vi "SP_OEE_REPORT_DAYWISE.vi"() -> ()   [LabVIEW 2017]
uses:
  Controls/OE_screen_cluster.ctl
  <vilib>/addons/database/Connection.llb/Conn ObjectReference.ctl
  <vilib>/Utility/error.llb/DialogType.ctl
  <vilib>/addons/database/Connection.llb/DB Tools Open Connec (Path).vi
  <vilib>/addons/database/Connection.llb/Conn Execute.vi
  <vilib>/addons/database/Recordset.llb/Rec Fetch Recordset Data (R).vi
  <vilib>/addons/database/Recordset.llb/Rec Destroy - Connection.vi
  <vilib>/addons/database/NI_Database_API.lvlib
panel:
  in  "Tab Control 2":enum32{"Calculations", "Product Time"}(tab)
  out "AT time (Min)":i32
  out "Net Avai time (Min)":i32
  out "Standard DT (Min)":i32
  out "Downtime":u32
  out "Run Time":u32
  out "A Rate %":i32
  out "Parts per hours":i32
  out "CT":dbl format="%.2f"
  out "Actual Production / Total Quantity":u32
  out "Expected Run Time":sgl
  out "P Rate %":sgl format="%#.2g"
  out "OK Count":u32
  out "Rejection Count":u32
  out "Quality %":u32
  out "Select Product":string
  out "Start time":timestamp=timestamp(3772871939 s since 1904-01-01) format="%<%.X \n%x>T"
  out "End Time":timestamp=timestamp(3772871939 s since 1904-01-01) format="%<%.X \n%x>T"
  out "Split DT time":u32[](array[numeric])
  out "appended path":path
  in  "Reset":bool
  out "appended path 4":path
  out "OEE %":dbl format="%.2f"
  out "breakdown out time":string[](array[string])
  out "breakdown in time":string[](array[string])
  out "data":string[][](array[string])
  in  "shift time selection":enum32{"Shift 1", "Shift 2"}(tab)
  in  "mislanius times shift 1":T1={"Lunch Time\nFrom"=timestamp(3772871904 s since 1904-01-01), "Lunch Time To"=timestamp(3772871909 s since 1904-01-01), "Tea Time\nFrom"=timestamp(3772871914 s since 1904-01-01), "Tea Time To"=timestamp(3772871912 s since 1904-01-01), "Clean Time\nFrom"=timestamp(3772871918 s since 1904-01-01), "Clean Time To"=timestamp(3772871916 s since 1904-01-01), "Meeting Time\nFrom"=timestamp(3772871920 s since 1904-01-01), "Meeting Time To"=timestamp(3772871922 s since 1904-01-01), "Dev/Other Time\n From"=timestamp(3772871924 s since 1904-01-01), "Dev/Other Time To"=timestamp(3771057526 s since 1904-01-01), "Meeting"=FALSE, "Dev/Other"=TRUE} {"Dev/Other Time To" format="%<%.X\n %x>T"; "Dev/Other Time\n From" format="%<%.X\n %x>T"; "Meeting Time To" format="%<%.X\n %x>T"; "Meeting Time\nFrom" format="%<%.X\n %x>T"; "Clean Time To" format="%<%.X\n %x>T"; "Clean Time\nFrom" format="%<%.X\n %x>T"; "Tea Time To" format="%<%.X\n %x>T"; "Tea Time\nFrom" format="%<%.X\n %x>T"; "Lunch Time To" format="%<%.X\n %x>T"; "Lunch Time\nFrom" format="%<%.X\n %x>T"}
  in  "mislanius times shift 2":T2={"Dinner Time\nFrom"=timestamp(3772871937 s since 1904-01-01), "To"=timestamp(3772871939 s since 1904-01-01), "Tea Time\nFrom"=timestamp(3772958341 s since 1904-01-01), "Tea Time To"=timestamp(3772958344 s since 1904-01-01), "Clean Time\nFrom"=timestamp(3772871947 s since 1904-01-01), "Clean Time To"=timestamp(3772871950 s since 1904-01-01), "Meeting Time\nFrom"=timestamp(3772871952 s since 1904-01-01), "Meeting Time To"=timestamp(3772871954 s since 1904-01-01), "Dev/Other Time\nFrom"=timestamp(3772871934 s since 1904-01-01), "Dev/Other Time To"=timestamp(3772871932 s since 1904-01-01), "Meeting"=TRUE, "Dev/Other"=TRUE} {"Dev/Other Time To" format="%<%.X \n%x>T"; "Dev/Other Time\nFrom" format="%<%.X \n%x>T"; "Meeting Time To" format="%<%.X \n%x>T"; "Meeting Time\nFrom" format="%<%.X \n%x>T"; "Clean Time To" format="%<%.X \n%x>T"; "Clean Time\nFrom" format="%<%.X \n%x>T"; "Tea Time To" format="%<%.X \n%x>T"; "Tea Time\nFrom" format="%<%.X \n%x>T"; "To" format="%<%.X \n%x>T"; "Dinner Time\nFrom" format="%<%.X \n%x>T"}
  out "time stamp":timestamp[](array[timestamp])
  out "Part Per Hour":i16
  out "Plan data":string[][](array[string])
  in  "Select Product":string(combo)
  in  "Generate Report":bool
  out "error out 2":errorcluster
  in  "error in.":errorcluster
  in  "Home":bool
  in  "Date":timestamp format="%<%Y-%m-%d>T"
  in  "Shift":string(combo)
  in  "Tab Control":enum32{"Statistical", "Graphical"}(tab)
  in  "Select Station":string(combo)
  # "Date"
  # "Safety"
  # "Logistic"
  # "Maintenance"
  # "Quality"
  # "Production"
  # "Total"
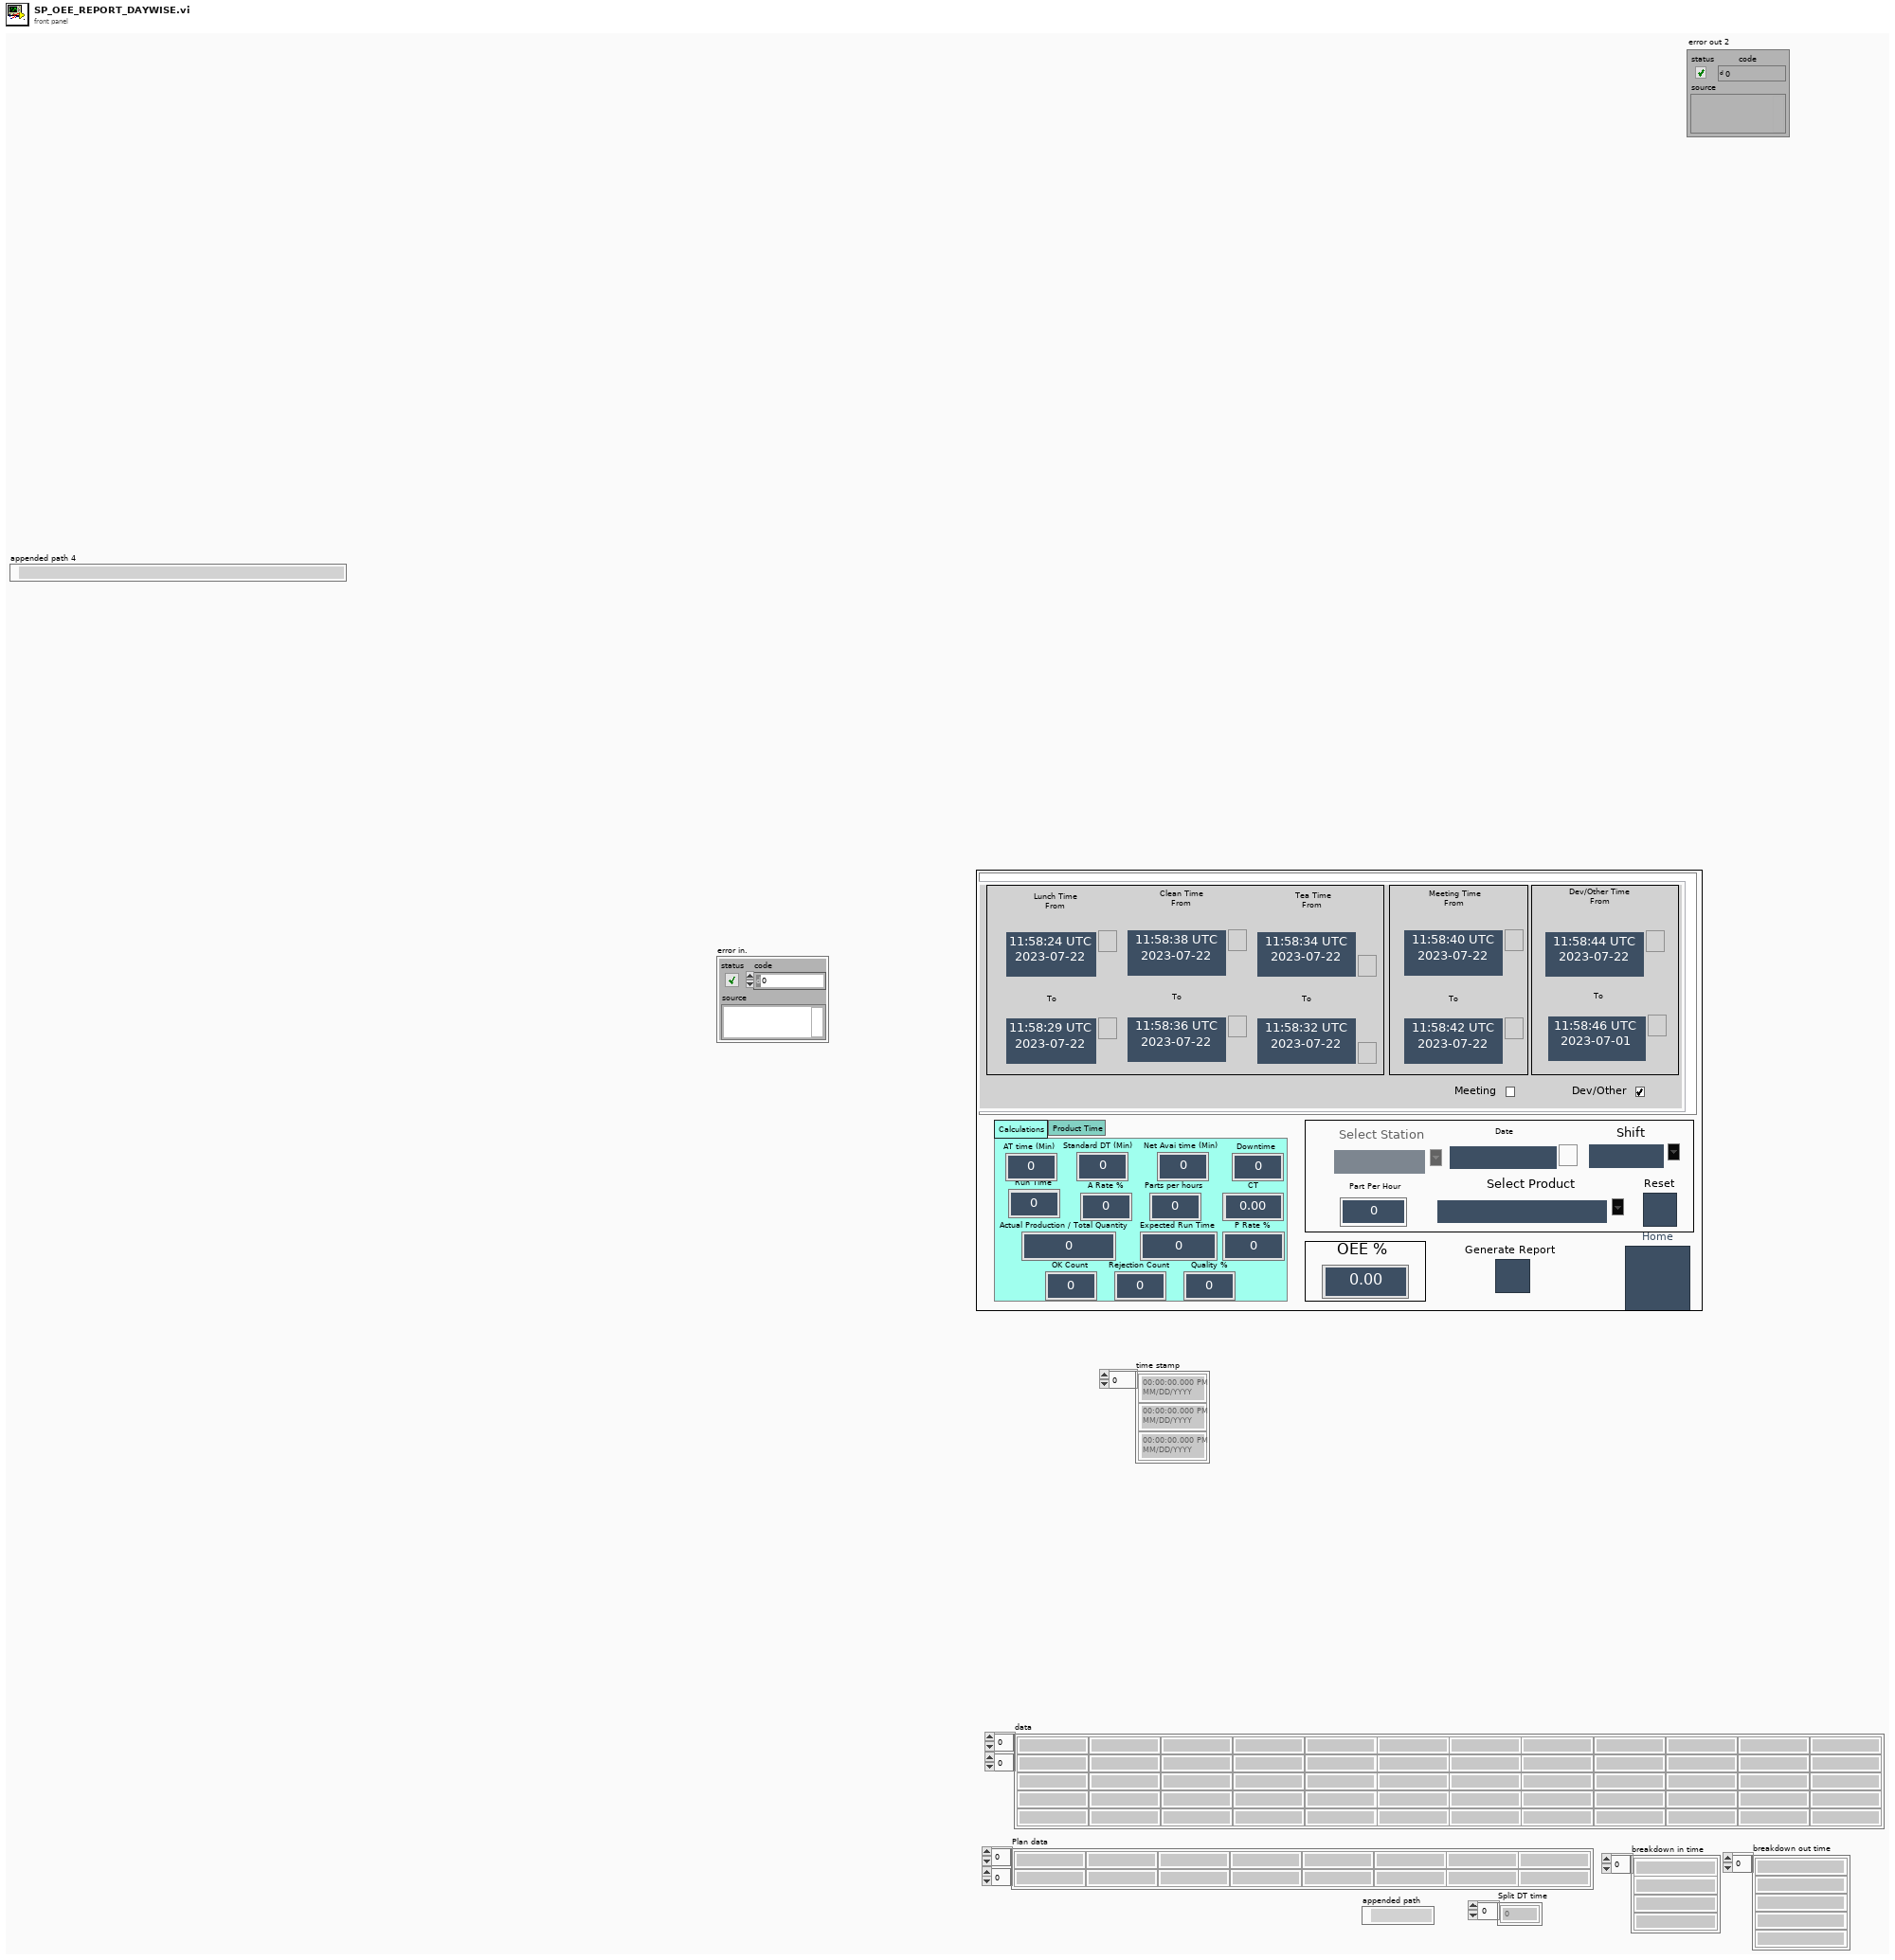
[diagram p1: front panel]
types:
  T1 = cluster{"Lunch Time\nFrom":timestamp, "Lunch Time To":timestamp, "Tea Time\nFrom":timestamp, "Tea Time To":timestamp, "Clean Time\nFrom":timestamp, "Clean Time To":timestamp, "Meeting Time\nFrom":timestamp, "Meeting Time To":timestamp, "Dev/Other Time\n From":timestamp, "Dev/Other Time To":timestamp, "Meeting":bool, "Dev/Other":bool}
  T2 = cluster{"Dinner Time\nFrom":timestamp, "To":timestamp, "Tea Time\nFrom":timestamp, "Tea Time To":timestamp, "Clean Time\nFrom":timestamp, "Clean Time To":timestamp, "Meeting Time\nFrom":timestamp, "Meeting Time To":timestamp, "Dev/Other Time\nFrom":timestamp, "Dev/Other Time To":timestamp, "Meeting":bool, "Dev/Other":bool}
  T3 = typedef "DialogType.ctl" = u16
  T4 = enum16{"open", "replace", "create", "open or create", "replace or create", "replace or create with confirmation"}
  T5 = cluster{"unsigned 64bit integer":u64, "unsigned 64bit integer 2":u64, "unsigned 64bit integer 3":u64, "unsigned 64bit integer 4":u64, "unsigned 64bit integer 5":u64, "unsigned 64bit integer 6":u64, "unsigned 64bit integer 7":u64, "unsigned 64bit integer 8":u64, "unsigned 64bit integer 9":u64, "unsigned 64bit integer 10":u64, "Meeting":bool, "Dev/other 1":bool, "unsigned 64bit integer 11":u64, "unsigned 64bit integer 12":u64, "unsigned 64bit integer 13":u64, "unsigned 64bit integer 14":u64, "unsigned 64bit integer 15":u64, "unsigned 64bit integer 16":u64, "unsigned 64bit integer 17":u64, "unsigned 64bit integer 18":u64, "unsigned 64bit integer 19":u64, "unsigned 64bit integer 20":u64, "Meeting 2":bool, "Dev/other 2":bool}
  T6 = enum8{"Enabled", "Disabled", "Disabled and Grayed Out"}
  T7 = typedef "OE_screen_cluster.ctl" = cluster{"connection reference":T8, "Net Avai time (Min)":i32, "pLAN dATE datA":string[][], "Data by plan date, shift, product":string[][], "BreakDownd Data":string[][], "Raw rejection Data":string[][], "mislanius times shift 1":cluster{"Lunch Time From":timestamp, "Lunch Time To":timestamp, "Tea Time From":timestamp, "Tea Time To":timestamp, "Clean Time From":timestamp, "Clean Time To":timestamp, "Meeting Time From":timestamp, "Meeting Time To":timestamp, "Dev/Other Time From":timestamp, "Dev/Other Time To":timestamp, "Meeting":bool, "Dev/Other":bool}, "mislanius times shift 2":cluster{"Lunch Time From":timestamp, "Lunch Time To":timestamp, "Tea Time From":timestamp, "Tea Time To":timestamp, "Clean Time From":timestamp, "Clean Time To":timestamp, "Meeting Time From":timestamp, "Meeting Time To":timestamp, "Dev/Other Time From":timestamp, "Dev/Other Time To":timestamp, "Meeting":bool, "Dev/Other":bool}}
  T8 = typedef "NI_Database_API.lvlib/Conn ObjectReference.ctl" = refnum<k1>
  T9 = enum32{"invalid app kind", "Development System", "Run Time System", "Student Edition", "Embedded LabVIEW", "Evaluation", "Custom"}
  T10 = typedef "NI_Database_API.lvlib/Rec ObjectReference.ctl" = refnum<k1>
  T11 = cluster{"delimiter (Tab)":string, "String":string}[]
  T12 = cluster{"Actual Production / Total Quantity":u32, "Part Per Hour":i16, "Rejection Count":u32}
  T13 = cluster{"Lunch Time From":timestamp, "Lunch Time To":timestamp, "Tea Time From":timestamp, "Tea Time To":timestamp, "Clean Time From":timestamp, "Clean Time To":timestamp, "Meeting Time From":timestamp, "Meeting Time To":timestamp, "Dev/Other Time From":timestamp, "Dev/Other Time To":timestamp, "Meeting":bool, "Dev/Other":bool}
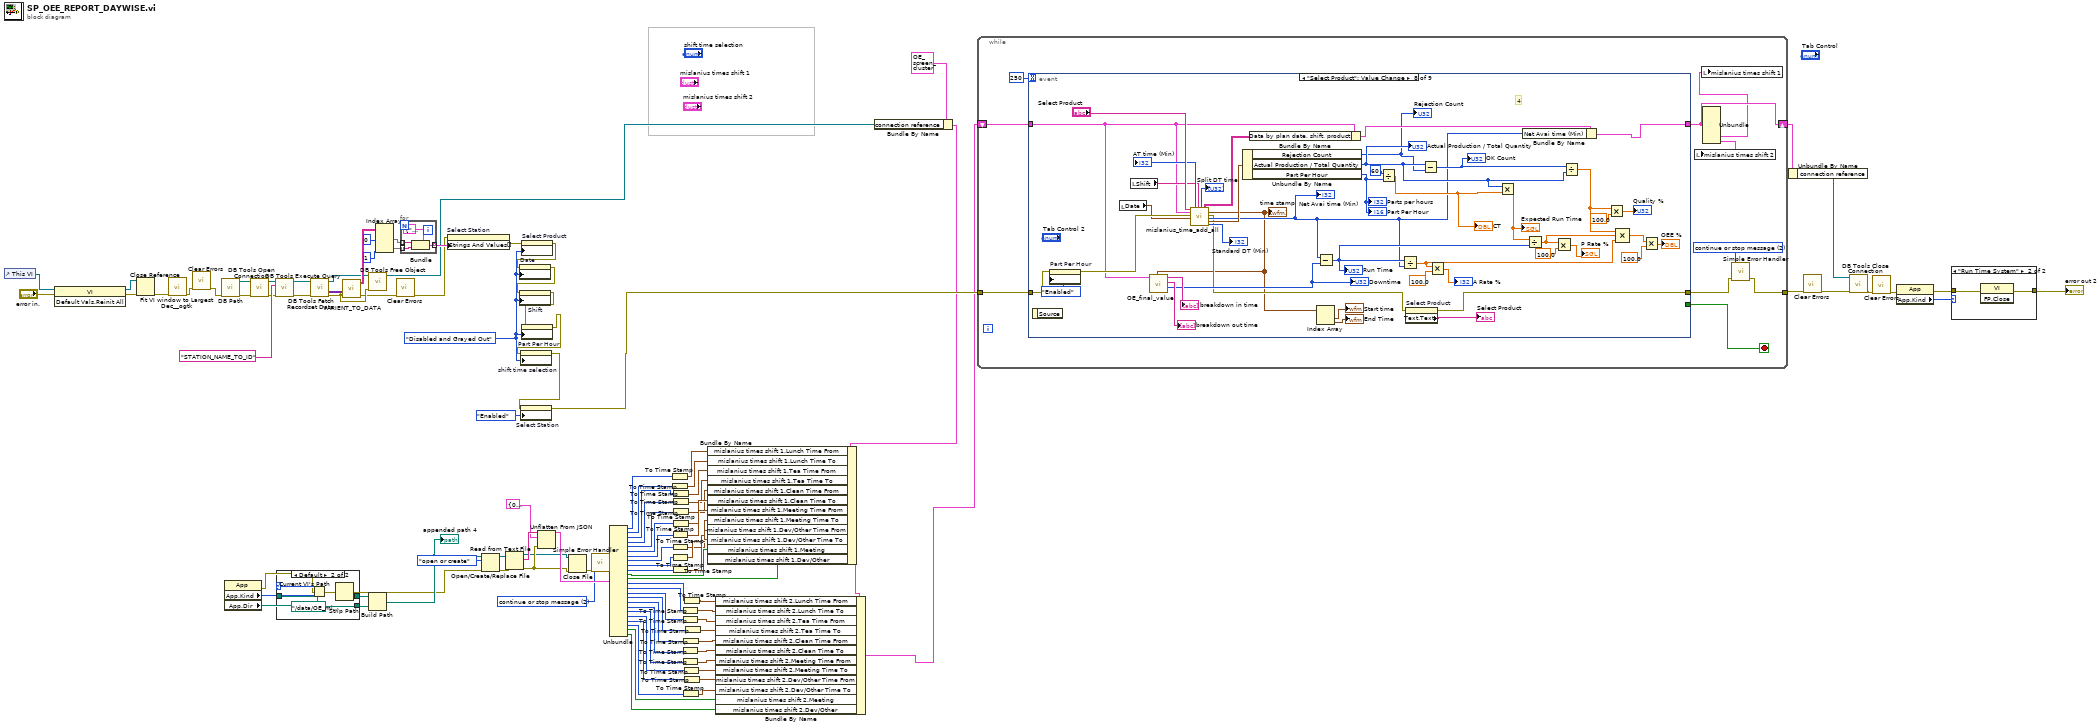
[diagram p0: block diagram]
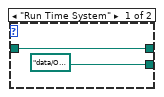
[diagram p2: hidden frame]
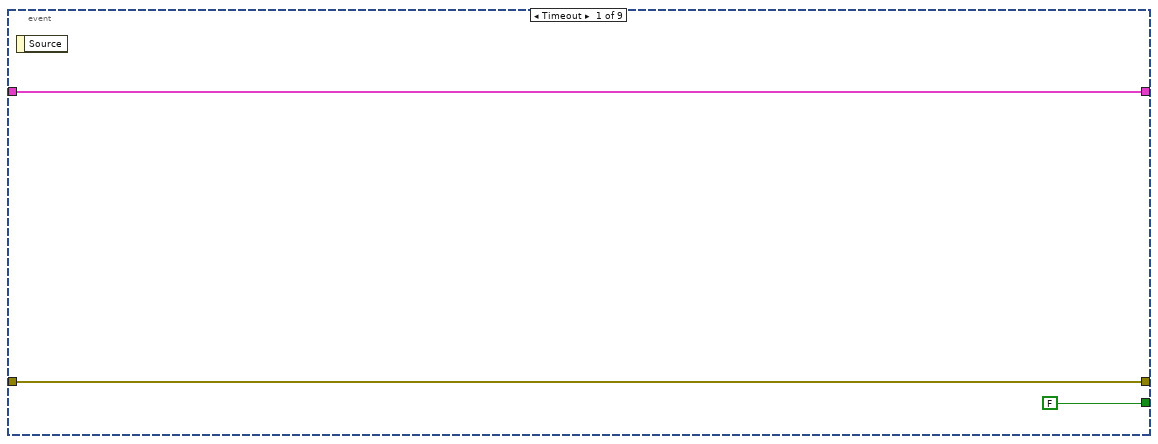
[diagram p4: hidden frame]
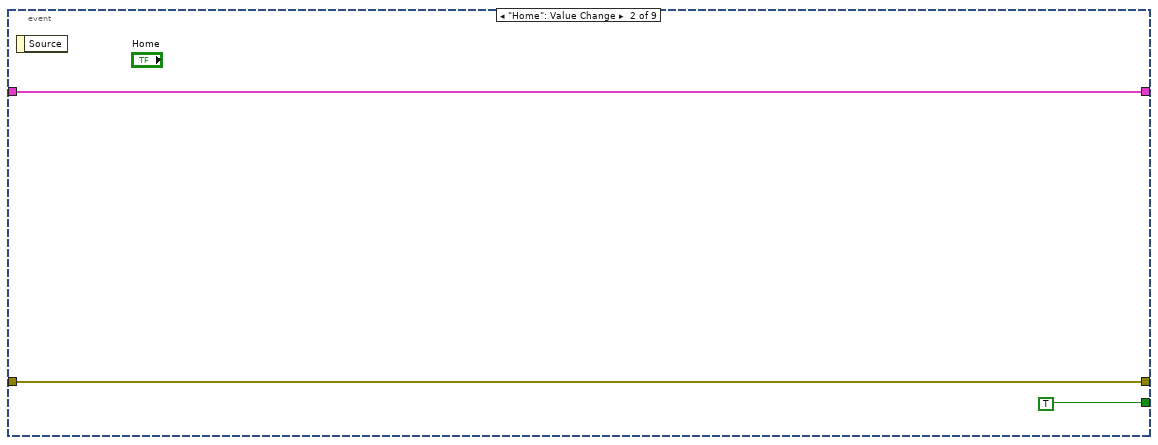
[diagram p5: hidden frame]
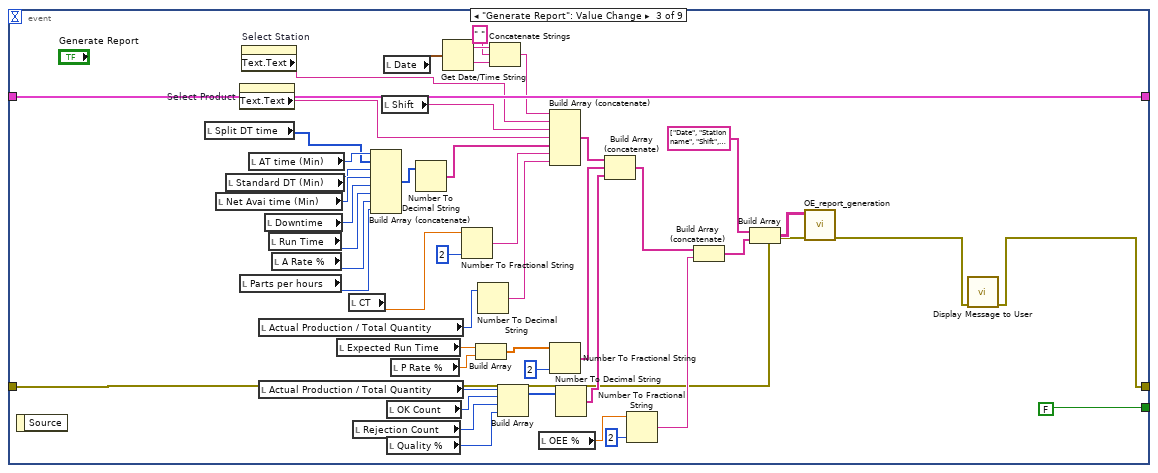
[diagram p6: hidden frame]
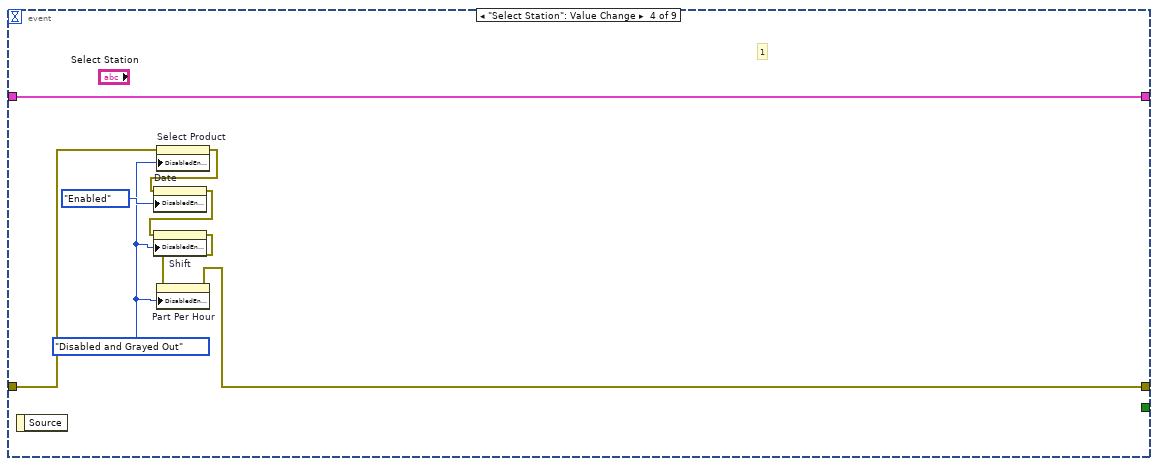
[diagram p7: hidden frame]
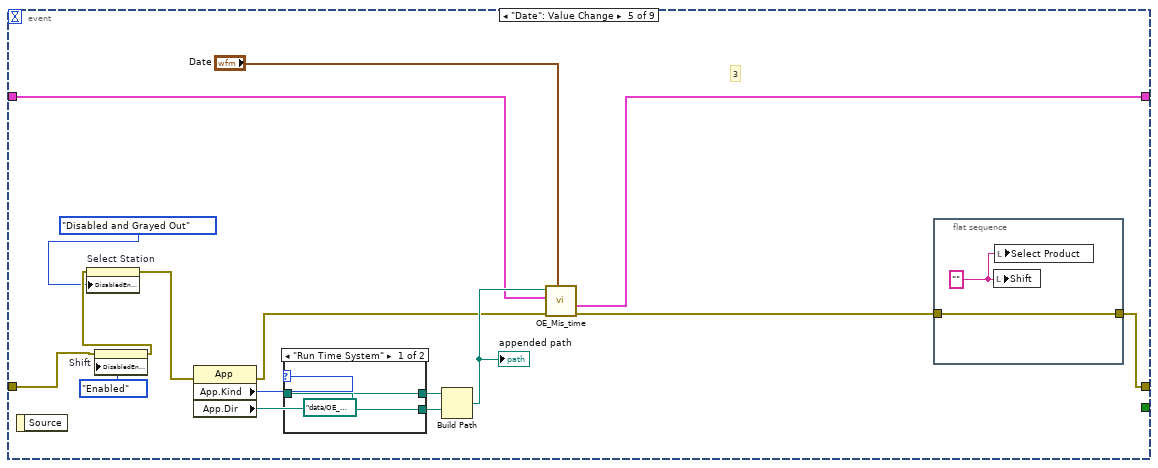
[diagram p8: hidden frame]
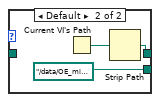
[diagram p9: hidden frame]
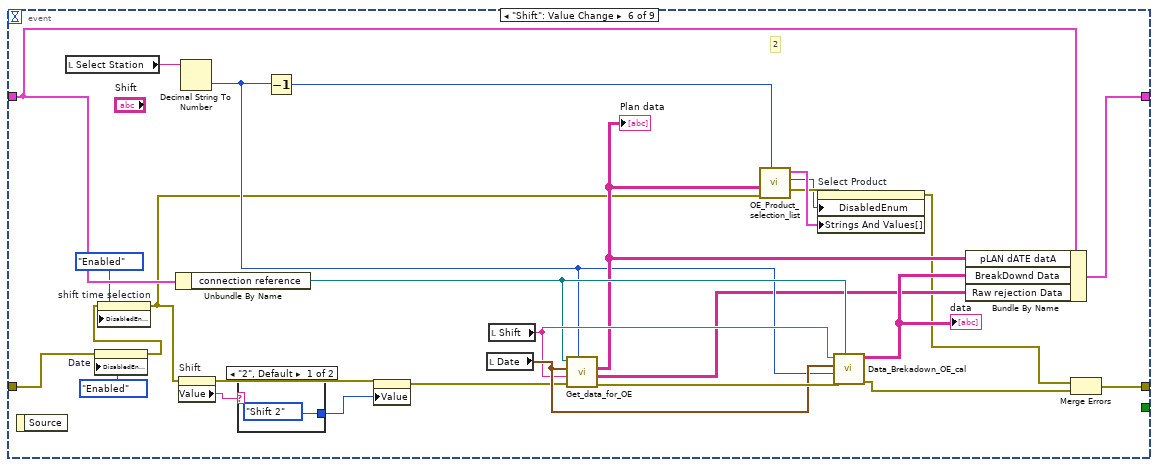
[diagram p10: hidden frame]
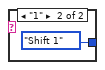
[diagram p11: hidden frame]
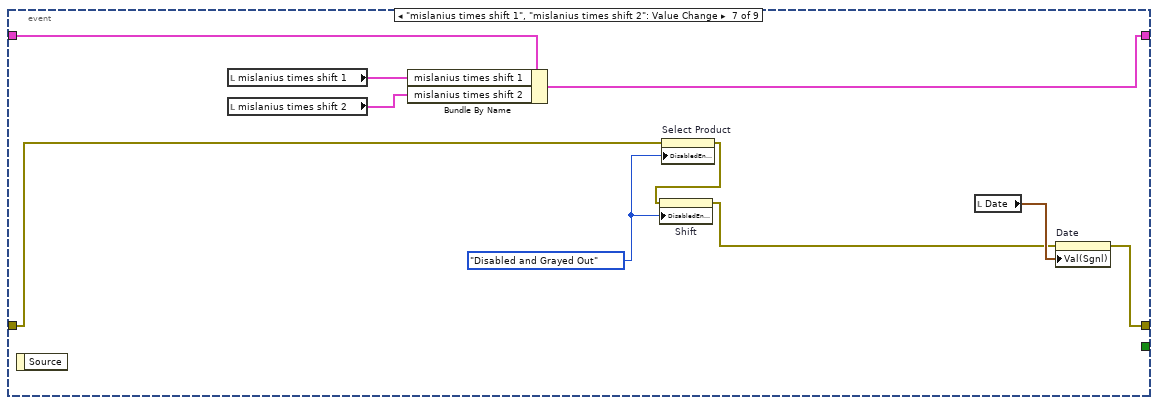
[diagram p12: hidden frame]
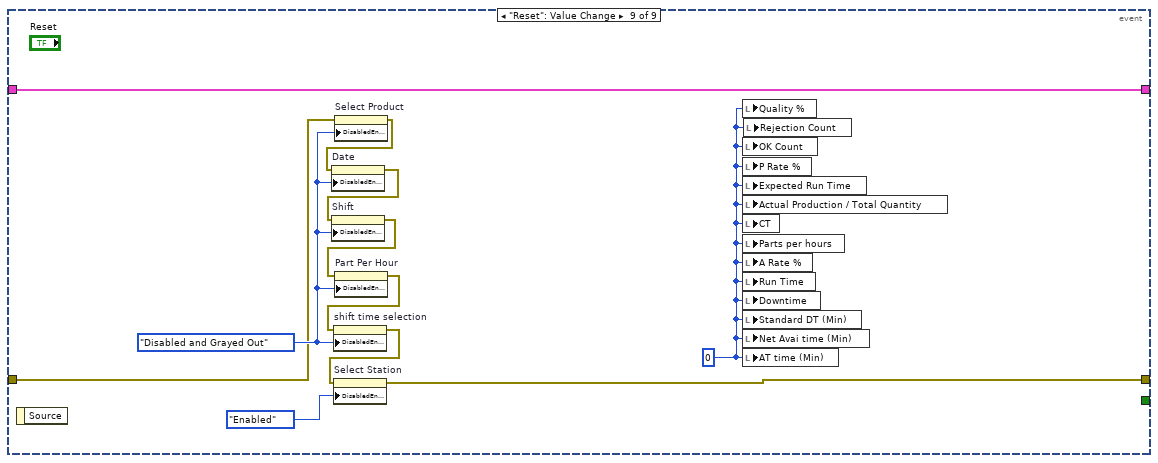
[diagram p13: hidden frame]
diagram:
  w6 = T3 2 items=["no dialog", "OK message", "continue or stop message", "OK message + warnings", "continue/stop + warnings"] ("type of dialog (OK msg:1)")
  w65 = T6."Disabled and Grayed Out" ("Disabled")
  n1 = control-ref of="This VI"() -> (w103:refnum<vi>)
  n2 = invoke class="VI" method="Default Vals.Reinit All"(reference=w103, error in="error in.") -> (reference out=w105:refnum<vi>, error out=w104:errorcluster)  [unwired: 1 in, 1 out]
  n3 = Close Reference(reference=w105, error in (no error)=w104) -> (error out=w5:errorcluster)
  n4 = call <userlib>:"Fit VI window to Largest Dec__ogtk.vi"("error in (no error)"=w5) -> ("error out"=w4:errorcluster)  [unwired: 5 in, 1 out]
  n5 = call <vilib>:"Clear Errors.vi"("error in (no error)"=w4) -> ("error out"=w3:errorcluster)  [unwired: 5 in, 1 out]
  n6 = call "DB Path.vi"("error in"=w3) -> ("error out"=w106:errorcluster, "DB Path"=w107:path)  [unwired: 9 in]
  n7 = property class="App"() -> (error out=w13:errorcluster, "App.Kind"=w70:T9, "App.Dir"=w71:path)  [unwired: 2 in, 1 out]
  n8 = call-poly <vilib>:"DB Tools Open Connection.vi"("error in (no error)"=w106, "connection information"=w107) -> ("error out"=w93:errorcluster, "connection reference"=w80:T8)  [unwired: 6 in]
  n9 = call-poly <vilib>:"DB Tools Execute Query.vi"("error in (no error)"=w93, "SQL query"="STATION_NAME_TO_ID", "connection reference"=w80) -> ("error out"=w101:errorcluster, "recordset reference"=w102:T10)  [unwired: 5 in]
  n10 = case shown="Default" w70 {
    tunnel: w71 -> [w110 _]
    tunnel: [path "data/OE_mis_time.txt" ("path") path "../data/OE_mis_time.txt" ("path")] -> w73
    tunnel: [w110 w112] -> w74
    frame "Run Time System" {
    }
    frame Default {
      n11 = Current VI's Path() -> (path=w113:path)
      n12 = Strip Path(path=w113) -> (stripped path=w112:path)  [unwired: 1 out]
    }
  }
  n13 = call-poly <vilib>:"DB Tools Fetch Recordset Data.vi"("error in (no error)"=w101, "recordset reference"=w102) -> ("error out"=w95:errorcluster, "recordset data"=w99:variant[][], "recordset reference out"=w81:T10)  [unwired: 3 in]
  n14 = call "VARIENT_TO_DATA.vi"("data"=w99, "error in (no error)"=w95) -> ("Table"=w96:string[][], "error out"=w94:errorcluster)  [unwired: 7 in]
  n15 = Build Path(base path=w74, name or relative path=w73) -> (appended path=w72:path)
  "appended path 4" <- w72
  n16 = call-poly <vilib>:"DB Tools Free Object.vi"("error in (no error)"=w95, "recordset reference"=w81) -> ("connection reference"=w79:T8)  [unwired: 8 in, 1 out]
  n17 = Index Array(array=w96, index (col) #1=0 ("index (row)"), index (col) #2=1 ("index (col)")) -> (element #1=w92:string[], element #2=w91:string[])  [unwired: 2 in]
  n18 = call <vilib>:"Clear Errors.vi"("error in (no error)"=w94) -> ("error out"=w89:errorcluster)  [unwired: 5 in, 1 out]
  n19 = for {
    tunnel: w92 -> [w117] mode=indexing
    tunnel: w91 -> [w116] mode=indexing
    tunnel: [w114] -> w90 mode=indexing
    n20 = Bundle(cluster=cluster{"String":string, "Value":string} {"String"="", "Value"=""}, "String"=w117, "Value"=w116) -> (w114:cluster{"String":string, "Value":string})
  }
  n21 = property on="Select Station" class="CmbBox"(error in=w89, "Strings And Values[]"=w90) -> (error out=w77:errorcluster)  [unwired: 1 in, 1 out]
  n22 = Open/Create/Replace File(file path (use dialog)=w72, error in=w13, operation (0:open)=T4."open or create") -> (refnum out=w69:refnum<file>, error out=w68:errorcluster)  [unwired: 3 in, 1 out]
  n23 = Read from Text File(file (use dialog)=w69, error in=w68) -> (refnum out=w9:refnum<file>, text=w12:string, error out=w10:errorcluster)  [unwired: 2 in, 1 out]
  n24 = property on="Select Product" class="CmbBox"(error in=w77, "DisabledEnum"=w65) -> (error out=w76:errorcluster)  [unwired: 1 in, 1 out]
  n25 = property on="Date" class="AbsTime (strict)"(error in=w76, "DisabledEnum"=w65) -> (error out=w78:errorcluster)  [unwired: 1 in, 1 out]
  n26 = property on="Shift" class="CmbBox"(error in=w78, "DisabledEnum"=w65) -> (error out=w75:errorcluster)  [unwired: 1 in, 1 out]
  n27 = property on="Part Per Hour" class="DigNum (strict)"(error in=w75, "DisabledEnum"=w65) -> (error out=w66:errorcluster)  [unwired: 1 in, 1 out]
  n28 = property on="shift time selection" class="TabCtl (strict)"(error in=w66, "DisabledEnum"=w65) -> (error out=w64:errorcluster)  [unwired: 1 in, 1 out]
  n29 = property on="Select Station" class="CmbBox"(error in=w64, "DisabledEnum"=T6."Enabled" ("Disabled")) -> (error out=w63:errorcluster)  [unwired: 1 in, 1 out]
  n30 = Unflatten From JSON(JSON string=w12, type and defaults=T5 {"unsigned 64bit integer"=0, "unsigned 64bit integer 2"=0, "unsigned 64bit integer 3"=0, "unsigned 64bit integer 4"=0, "unsigned 64bit integer 5"=0, "unsigned 64bit integer 6"=0, "unsigned 64bit integer 7"=0, "unsigned 64bit integer 8"=0, "unsigned 64bit integer 9"=0, "unsigned 64bit integer 10"=0, "Meeting"=FALSE, "Dev/other 1"=FALSE, "unsigned 64bit integer 11"=0, "unsigned 64bit integer 12"=0, "unsigned 64bit integer 13"=0, "unsigned 64bit integer 14"=0, "unsigned 64bit integer 15"=0, "unsigned 64bit integer 16"=0, "unsigned 64bit integer 17"=0, "unsigned 64bit integer 18"=0, "unsigned 64bit integer 19"=0, "unsigned 64bit integer 20"=0, "Meeting 2"=FALSE, "Dev/other 2"=FALSE} ("input cluster"), error in (no error)=w10) -> (value=w51:T5)  [unwired: 4 in, 1 out]
  n31 = Close File(refnum=w9, error in=w10) -> (error out=w7:errorcluster)  [unwired: 1 out]
  n32 = call <vilib>:"Simple Error Handler.vi"("type of dialog (OK msg:1)"=w6, "error in (no error)"=w7) -> ()  [unwired: 3 in, 5 out]
  n33 = Unbundle(w51) -> ("unsigned 64bit integer"=w36:u64, "unsigned 64bit integer 2"=w35:u64, "unsigned 64bit integer 3"=w34:u64, "unsigned 64bit integer 4"=w33:u64, "unsigned 64bit integer 5"=w32:u64, "unsigned 64bit integer 6"=w31:u64, "unsigned 64bit integer 7"=w30:u64, "unsigned 64bit integer 8"=w29:u64, "unsigned 64bit integer 9"=w28:u64, "unsigned 64bit integer 10"=w27:u64, "Meeting"=w38:bool, "Dev/other 1"=w37:bool, "unsigned 64bit integer 11"=w16:u64, "unsigned 64bit integer 12"=w17:u64, "unsigned 64bit integer 13"=w18:u64, "unsigned 64bit integer 14"=w19:u64, "unsigned 64bit integer 15"=w20:u64, "unsigned 64bit integer 16"=w21:u64, "unsigned 64bit integer 17"=w22:u64, "unsigned 64bit integer 18"=w23:u64, "unsigned 64bit integer 19"=w24:u64, "unsigned 64bit integer 20"=w25:u64, "Meeting 2"=w26:bool, "Dev/other 2"=w39:bool)
  n34 = To Time Stamp(1:w36) -> (0:w52:timestamp)
  n35 = To Time Stamp(1:w35) -> (0:w53:timestamp)
  n36 = To Time Stamp(1:w30) -> (0:w58:timestamp)
  n37 = To Time Stamp(1:w29) -> (0:w59:timestamp)
  n38 = To Time Stamp(1:w28) -> (0:w60:timestamp)
  n39 = To Time Stamp(1:w27) -> (0:w61:timestamp)
  n40 = To Time Stamp(1:w34) -> (0:w54:timestamp)
  n41 = To Time Stamp(1:w33) -> (0:w55:timestamp)
  n42 = To Time Stamp(1:w32) -> (0:w56:timestamp)
  n43 = To Time Stamp(1:w31) -> (0:w57:timestamp)
  n44 = To Time Stamp(1:w17) -> (0:w49:timestamp)
  n45 = To Time Stamp(1:w18) -> (0:w48:timestamp)
  n46 = To Time Stamp(1:w21) -> (0:w45:timestamp)
  n47 = To Time Stamp(1:w22) -> (0:w44:timestamp)
  n48 = To Time Stamp(1:w20) -> (0:w46:timestamp)
  n49 = To Time Stamp(1:w25) -> (0:w41:timestamp)
  n50 = To Time Stamp(1:w23) -> (0:w43:timestamp)
  n51 = To Time Stamp(1:w16) -> (0:w50:timestamp)
  n52 = To Time Stamp(1:w24) -> (0:w42:timestamp)
  n53 = To Time Stamp(1:w19) -> (0:w47:timestamp)
  n54 = Bundle By Name(cluster=T7 {"connection reference"=refnum, "Net Avai time (Min)"=0, "pLAN dATE datA"=[], "Data by plan date, shift, product"=[], "BreakDownd Data"=[], "Raw rejection Data"=[], "mislanius times shift 1"={"Lunch Time From"=timestamp(0 s since 1904-01-01), "Lunch Time To"=timestamp(0 s since 1904-01-01), "Tea Time From"=timestamp(0 s since 1904-01-01), "Tea Time To"=timestamp(0 s since 1904-01-01), "Clean Time From"=timestamp(0 s since 1904-01-01), "Clean Time To"=timestamp(0 s since 1904-01-01), "Meeting Time From"=timestamp(0 s since 1904-01-01), "Meeting Time To"=timestamp(0 s since 1904-01-01), "Dev/Other Time From"=timestamp(0 s since 1904-01-01), "Dev/Other Time To"=timestamp(0 s since 1904-01-01), "Meeting"=FALSE, "Dev/Other"=TRUE}, "mislanius times shift 2"={"Lunch Time From"=timestamp(0 s since 1904-01-01), "Lunch Time To"=timestamp(0 s since 1904-01-01), "Tea Time From"=timestamp(0 s since 1904-01-01), "Tea Time To"=timestamp(0 s since 1904-01-01), "Clean Time From"=timestamp(0 s since 1904-01-01), "Clean Time To"=timestamp(0 s since 1904-01-01), "Meeting Time From"=timestamp(0 s since 1904-01-01), "Meeting Time To"=timestamp(0 s since 1904-01-01), "Dev/Other Time From"=timestamp(0 s since 1904-01-01), "Dev/Other Time To"=timestamp(0 s since 1904-01-01), "Meeting"=FALSE, "Dev/Other"=TRUE}}, "connection reference"=w79) -> (w15:T7)
  n55 = Bundle By Name(cluster=w15, "mislanius times shift 1.Lunch Time From"=w52, "mislanius times shift 1.Lunch Time To"=w53, "mislanius times shift 1.Tea Time From"=w54, "mislanius times shift 1.Tea Time To"=w55, "mislanius times shift 1.Clean Time From"=w56, "mislanius times shift 1.Clean Time To"=w57, "mislanius times shift 1.Meeting Time From"=w58, "mislanius times shift 1.Meeting Time To"=w59, "mislanius times shift 1.Dev/Other Time From"=w60, "mislanius times shift 1.Dev/Other Time To"=w61, "mislanius times shift 1.Meeting"=w38, "mislanius times shift 1.Dev/Other"=w37) -> (w40:T7)
  n56 = Bundle By Name(cluster=w40, "mislanius times shift 2.Lunch Time From"=w50, "mislanius times shift 2.Lunch Time To"=w49, "mislanius times shift 2.Tea Time From"=w48, "mislanius times shift 2.Tea Time To"=w47, "mislanius times shift 2.Clean Time From"=w46, "mislanius times shift 2.Clean Time To"=w45, "mislanius times shift 2.Meeting Time From"=w44, "mislanius times shift 2.Meeting Time To"=w43, "mislanius times shift 2.Dev/Other Time From"=w42, "mislanius times shift 2.Dev/Other Time To"=w41, "mislanius times shift 2.Meeting"=w26, "mislanius times shift 2.Dev/Other"=w39) -> (w14:T7)
  n57 = while {
    tunnel: w63 -> [w127]
    shift-right: [w125] -> w83
    shift-left: w14 -> [w126]
    tunnel: [w119] -> w2
    stop <- w124 stop-if-true
    w118 = T3 2 items=["no dialog", "OK message", "continue or stop message", "OK message + warnings", "continue/stop + warnings"] ("type of dialog (OK msg:1)")
    n58 = event shown="[7] \"Select Product\": Value Change" {
      selector: _ -> [_ _ _ _ _ _ _ _ _]
      dyn-events: _ -> [_ _ _ _ _ _ _ _ _]
      timeout: 250 -> [_ _ _ _ _ _ _ _ _]
      tunnel: w127 -> [w129 w131 w140 w186 w203 w237 w241 w293 w297]
      tunnel: [w130 w132 w179 w188 w195 w231 w249 w291 w305] -> w125
      tunnel: w126 -> [w130 w132 w179 w188 w196 w232 w250 w263 w305]
      tunnel: [FALSE TRUE FALSE _ _ _ _ _ _] -> w124
      tunnel: [w129 w131 w141 w185 w189 w216 w246 w253 w296] -> w120
      event Timeout {
        n59 = event-data() -> ()  [unwired: 1 in, 1 out]
      }
      event "Home": Value Change {
        n60 = event-data() -> ()  [unwired: 1 in, 1 out]
      }
      event "Generate Report": Value Change {
        n61 = event-data() -> ()  [unwired: 1 in, 1 out]
        n62 = local read "Split DT time"() -> (w136:u32[])
        n63 = local read "Net Avai time (Min)"() -> (w172:i32)
        n64 = local read "Standard DT (Min)"() -> (w171:i32)
        n65 = property on="Select Product" class="CmbBox"() -> ("Text.Text"=w134:string)  [unwired: 2 in, 2 out]
        n66 = local read "Parts per hours"() -> (w166:i32)
        n67 = property on="Select Station" class="CmbBox"() -> ("Text.Text"=w135:string)  [unwired: 2 in, 2 out]
        n68 = local read "AT time (Min)"() -> (w137:i32)
        n69 = local read "Actual Production / Total Quantity"() -> (w161:u32)
        n70 = local read "Actual Production / Total Quantity"() -> (w154:u32)
        n71 = local read "Downtime"() -> (w169:u32)
        n72 = local read "Run Time"() -> (w168:u32)
        n73 = local read "A Rate %"() -> (w167:i32)
        n74 = local read "Expected Run Time"() -> (w159:sgl)
        n75 = local read "CT"() -> (w165:dbl)
        n76 = local read "Rejection Count"() -> (w152:u32)
        n77 = Build Array (concatenate)(w137, w136, w171, w172, w169, w168, w167, w166) -> (w170:u32[])
        n78 = local read "Shift"() -> (w173:string)
        n79 = local read "Date"() -> (w178:timestamp)
        n80 = local read "OK Count"() -> (w153:u32)
        n81 = local read "Quality %"() -> (w149:u32)
        n82 = local read "P Rate %"() -> (w158:sgl)
        n83 = Number To Decimal String(number=w170) -> (decimal integer string=w138:string[])  [unwired: 1 in]
        n84 = Get Date/Time String(seconds (now)=w178) -> (date string=w177:string, time string=w176:string)  [unwired: 2 in]
        n85 = Number To Fractional String(number=w165, precision (6)=i16 2) -> (F-format string=w163:string)  [unwired: 2 in]
        n86 = Build Array(w159, w158) -> (w157:sgl[])
        n87 = Number To Decimal String(number=w161) -> (decimal integer string=w160:string)  [unwired: 1 in]
        n88 = Concatenate Strings(w177, " " ("string"), w176) -> (w174:string)
        n89 = Build Array(w154, w153, w152, w149) -> (w151:u32[])
        n90 = local read "OEE %"() -> (w147:dbl)
        n91 = Build Array (concatenate)(w174, w135, w173, w134, w138, w163, w160) -> (w156:string[])
        n92 = Number To Fractional String(number=w157, precision (6)=i16 2) -> (F-format string=w155:string[])  [unwired: 2 in]
        n93 = Number To Decimal String(number=w151) -> (decimal integer string=w150:string[])  [unwired: 1 in]
        n94 = Build Array (concatenate)(w156, w155, w150) -> (w145:string[])
        n95 = Number To Fractional String(number=w147, precision (6)=i16 2) -> (F-format string=w146:string)  [unwired: 2 in]
        n96 = Build Array (concatenate)(w145, w146) -> (w144:string[])
        n97 = Build Array(string[] ["Date", "Station name", "Shift", "Select Product", "AT Time (min)", "Lunch Time", "Tea Time", "Cleaning Time", "Meeting Time", "Dev/Other Time", "Standard Time", "Net Available Time", "DOWNTIME", "RUN Time", "A RATE %", "Parts Per Hour", "CT %", "Actual Production", "Expected Run Time", "P RATE %", "Total Quantity", "OK Count", "Rejection Count", "Quality %", "OEE %"] ("Column Header Strings[]"), w144) -> (w143:string[][])
        n98 = call "OE_report_generation.vi"("error in (no error)"=w140, "Column Header and data"=w143) -> ("error out"=w142:errorcluster)  [unwired: 9 in]
        n99 = call "Display Message to User"("error in (no error)"=w142) -> ("error out"=w141:errorcluster)  [unwired: 9 in, 1 out]
      }
      event "Select Station": Value Change {
        w181 = T6."Disabled and Grayed Out" ("Disabled")
        # "1"
        n100 = event-data() -> ()  [unwired: 1 in, 1 out]
        n101 = property on="Select Product" class="CmbBox"(error in=w186, "DisabledEnum"=w181) -> (error out=w183:errorcluster)  [unwired: 1 in, 1 out]
        n102 = property on="Date" class="AbsTime (strict)"(error in=w183, "DisabledEnum"=T6."Enabled" ("Disabled")) -> (error out=w182:errorcluster)  [unwired: 1 in, 1 out]
        n103 = property on="Shift" class="CmbBox"(error in=w182, "DisabledEnum"=w181) -> (error out=w187:errorcluster)  [unwired: 1 in, 1 out]
        n104 = property on="Part Per Hour" class="DigNum (strict)"(error in=w187, "DisabledEnum"=w181) -> (error out=w185:errorcluster)  [unwired: 1 in, 1 out]
      }
      event "Date": Value Change {
        # "3"
        n105 = event-data() -> ()  [unwired: 1 in, 1 out]
        n106 = property on="Shift" class="CmbBox"(error in=w203, "DisabledEnum"=T6."Enabled" ("Disabled")) -> (error out=w194:errorcluster)  [unwired: 1 in, 1 out]
        n107 = property on="Select Station" class="CmbBox"(error in=w194, "DisabledEnum"=T6."Disabled and Grayed Out" ("Disabled")) -> (error out=w193:errorcluster)  [unwired: 1 in, 1 out]
        n108 = property class="App"(error in=w193) -> (error out=w197:errorcluster, "App.Kind"=w202:T9, "App.Dir"=w201:path)  [unwired: 1 in, 1 out]
        n109 = case shown="\"Run Time System\"" w202 {
          tunnel: w201 -> [w208 _]
          tunnel: [path "data/OE_mis_time.txt" ("path") path "../data/OE_mis_time.txt" ("path")] -> w199
          tunnel: [w208 w210] -> w198
          frame "Run Time System" {
          }
          frame Default {
            n110 = Current VI's Path() -> (path=w211:path)
            n111 = Strip Path(path=w211) -> (stripped path=w210:path)  [unwired: 1 out]
          }
        }
        n112 = Build Path(base path=w198, name or relative path=w199) -> (appended path=w200:path)
        "appended path" <- w200
        n113 = call "OE_Mis_time.vi"("Seelected date"="Date", "error in (no error)"=w197, "Cluster in"=w196, "appended path"=w200) -> ("error out"=w190:errorcluster, "Cluster out"=w195:T7)  [unwired: 6 in]
        n114 = flat-sequence {
          tunnel: [w205] -> w189
          tunnel: w190 -> [w205]
          frame #0 {
            w206 = ""
            n115 = local write "Shift"(w206) -> ()
            n116 = local write "Select Product"(w206) -> ()
          }
        }
      }
      event "Shift": Value Change {
        # "2"
        n117 = event-data() -> ()  [unwired: 1 in, 1 out]
        n118 = local read "Select Station"() -> (w236:string)
        n119 = property on="Date" class="AbsTime (strict)"(error in=w237, "DisabledEnum"=T6."Enabled" ("Disabled")) -> (error out=w215:errorcluster)  [unwired: 1 in, 1 out]
        n120 = property on="shift time selection" class="TabCtl (strict)"(error in=w215, "DisabledEnum"=T6."Enabled" ("Disabled")) -> (error out=w214:errorcluster)  [unwired: 1 in, 1 out]
        n121 = Unbundle By Name(w232) -> ("connection reference"=w227:T8)
        n122 = property on="Shift" class="CmbBox"(error in=w214) -> (error out=w234:errorcluster, "Value"=w233:string)  [unwired: 1 in, 1 out]
        n123 = Decimal String To Number(string=w236) -> (number=w220:i32)  [unwired: 2 in, 1 out]
        n124 = case shown="\"2\", Default" w233 {
          tunnel: [enum32{"Shift 1", "Shift 2"}."Shift 2" ("SHift mis time tab") enum32{"Shift 1", "Shift 2"}."Shift 1" ("SHift mis time tab")] -> w235
          frame "2", Default {
          }
          frame "1" {
          }
        }
        n125 = Decrement(x=w220) -> (x-1=w225:i32)
        n126 = property on="shift time selection" class="TabCtl (strict)"(error in=w234, "Value"=w235) -> (error out=w223:errorcluster)  [unwired: 1 in, 1 out]
        n127 = local read "Date"() -> (w229:timestamp)
        n128 = local read "Shift"() -> (w228:string)
        n129 = call "Get_data_for_OE.vi"("Station no."=w220, "error in (no error)"=w223, "Shift"=w228, "Date"=w229, "Refnum in"=w227) -> ("error out"=w230:errorcluster, "Rejected Product Data"=w219:string[][], "data"=w221:string[][])  [unwired: 3 in, 1 out]
        "Plan data" <- w221
        n130 = call "OE_Product_selection_list.vi"("Numeric"=w225, "error in (no error)"=w214, "Plan data"=w221) -> ("error out"=w222:errorcluster, "Disabled"=w212:T6, "Array out"=w224:T11)  [unwired: 6 in]
        n131 = property on="Select Product" class="CmbBox"(error in=w222, "DisabledEnum"=w212, "Strings And Values[]"=w224) -> (error out=w218:errorcluster)  [unwired: 1 in, 1 out]
        n132 = call "Data_Brekadown_OE_cal.vi"("Refnum in"=w227, "error in (no error)"=w230, "Station No"=w220, "Date"=w229, "Shift"=w228) -> ("error out"=w217:errorcluster, "Break_down_Data"=w226:string[][])  [unwired: 5 in]
        "data" <- w226
        n133 = Bundle By Name(cluster=w232, "pLAN dATE datA"=w221, "BreakDownd Data"=w226, "Raw rejection Data"=w219) -> (w231:T7)
        n134 = Merge Errors(w218, w217) -> (w216:errorcluster)
      }
      event "mislanius times shift 1", "mislanius times shift 2": Value Change {
        w242 = T6."Disabled and Grayed Out" ("Disabled")
        n135 = event-data() -> ()  [unwired: 1 in, 1 out]
        n136 = local read "mislanius times shift 1"() -> (w248:T1)
        n137 = local read "mislanius times shift 2"() -> (w247:T2)
        n138 = Bundle By Name(cluster=w250, "mislanius times shift 1"=w248, "mislanius times shift 2"=w247) -> (w249:T7)
        n139 = property on="Select Product" class="CmbBox"(error in=w241, "DisabledEnum"=w242) -> (error out=w243:errorcluster)  [unwired: 1 in, 1 out]
        n140 = property on="Shift" class="CmbBox"(error in=w243, "DisabledEnum"=w242) -> (error out=w244:errorcluster)  [unwired: 1 in, 1 out]
        n141 = local read "Date"() -> (w245:timestamp)
        n142 = property on="Date" class="AbsTime (strict)"(error in=w244, "Val(Sgnl)"=w245) -> (error out=w246:errorcluster)  [unwired: 1 in, 1 out]
      }
      event "Select Product": Value Change {
        # "4"
        n143 = event-data() -> ()  [unwired: 1 in, 1 out]
        n144 = property on="Part Per Hour" class="DigNum (strict)"(error in=w293, "DisabledEnum"=T6."Enabled" ("Disabled")) -> (error out=w270:errorcluster)  [unwired: 1 in, 1 out]
        n145 = local read "Date"() -> (w257:timestamp)
        n146 = local read "Shift"() -> (w269:string)
        n147 = call "mislanius_time_add_all.vi"("Select Product"="Select Product", "Cluster"=w263, "error in (no error)"=w270, "Date"=w257, "Shift"=w269) -> ("AT min"=→"AT time (Min)":i32, "Split DT time"=→"Split DT time":u32[], "Only select product and date and shift data"=w283:string[][], "1st and last cycle time stamp"=w251:timestamp[], "error out"=w254:errorcluster, "Net Available Time"=w261:u32, "output cluster"=w266:T12, "Total mis time"=→"Standard DT (Min)":i32)  [unwired: 7 in]
        "time stamp" <- w251
        "Net Avai time (Min)" <- w261
        n148 = call "OE_final_value.vi"("time stamp"=w251, "input cluster"=w263) -> ("Breakdown time"=w286:u32, "breakdown out time"=→"breakdown out time":string[], "breakdown in time"=→"breakdown in time":string[])  [unwired: 7 in]
        "Downtime" <- w286
        n149 = Unbundle By Name(w266) -> ("Rejection Count"=w262:u32, "Actual Production / Total Quantity"=w265:u32, "Part Per Hour"=w264:i16)
        "Part Per Hour" <- w264
        "Parts per hours" <- w264
        "Actual Production / Total Quantity" <- w265
        "Rejection Count" <- w262
        n150 = Bundle By Name(cluster=w263, "Data by plan date, shift, product"=w283) -> (w289:T7)
        n151 = Index Array(array=w251) -> (element #1=→"Start time":timestamp, element #2=→"End Time":timestamp)  [unwired: 2 in]
        n152 = Subtract(x=w261, y=w286) -> (x-y=w280:u32)
        "Run Time" <- w280
        n153 = Divide(x=i16 60, y=w264) -> (x/y=w282:dbl)
        "CT" <- w282
        n154 = Divide(x=w280, y=w261) -> (x/y=w258:dbl)
        n155 = property on="Select Product" class="CmbBox"(error in=w254) -> (error out=w253:errorcluster, "Text.Text"=→"Select Product":string)  [unwired: 1 in, 1 out]
        n156 = Subtract(x=w265, y=w262) -> (x-y=w279:u32)
        "OK Count" <- w279
        n157 = Multiply(x=w258, y=100.0) -> (x*y=→"A Rate %":dbl)
        n158 = Multiply(x=w265, y=w282) -> (x*y=w281:dbl)
        "Expected Run Time" <- w281
        n159 = Bundle By Name(cluster=w289, "Net Avai time (Min)"=w261) -> (w291:T7)
        n160 = Divide(x=w281, y=w280) -> (x/y=w260:dbl)
        n161 = Multiply(x=w260, y=100.0) -> (x*y=→"P Rate %":dbl)
        n162 = Divide(x=w279, y=w265) -> (x/y=w259:dbl)
        n163 = Multiply(x=w259, y=100.0) -> (x*y=→"Quality %":dbl)
        n164 = Compound Arithmetic op=MULTIPLY(w259, w260, w258) -> (w272:dbl)
        n165 = Multiply(x=w272, y=100.0) -> (x*y=→"OEE %":dbl)
      }
      event "Reset": Value Change {
        w295 = 0
        w302 = T6."Disabled and Grayed Out" ("Disabled")
        n166 = event-data() -> ()  [unwired: 1 in, 1 out]
        n167 = property on="Select Product" class="CmbBox"(error in=w297, "DisabledEnum"=w302) -> (error out=w299:errorcluster)  [unwired: 1 in, 1 out]
        n168 = property on="Date" class="AbsTime (strict)"(error in=w299, "DisabledEnum"=w302) -> (error out=w298:errorcluster)  [unwired: 1 in, 1 out]
        n169 = property on="Shift" class="CmbBox"(error in=w298, "DisabledEnum"=w302) -> (error out=w300:errorcluster)  [unwired: 1 in, 1 out]
        n170 = property on="Part Per Hour" class="DigNum (strict)"(error in=w300, "DisabledEnum"=w302) -> (error out=w301:errorcluster)  [unwired: 1 in, 1 out]
        n171 = property on="shift time selection" class="TabCtl (strict)"(error in=w301, "DisabledEnum"=w302) -> (error out=w303:errorcluster)  [unwired: 1 in, 1 out]
        n172 = property on="Select Station" class="CmbBox"(error in=w303, "DisabledEnum"=T6."Enabled" ("Disabled")) -> (error out=w296:errorcluster)  [unwired: 1 in, 1 out]
        n173 = local write "Quality %"(w295) -> ()
        n174 = local write "OK Count"(w295) -> ()
        n175 = local write "P Rate %"(w295) -> ()
        n176 = local write "Expected Run Time"(w295) -> ()
        n177 = local write "Actual Production / Total Quantity"(w295) -> ()
        n178 = local write "CT"(w295) -> ()
        n179 = local write "Parts per hours"(w295) -> ()
        n180 = local write "A Rate %"(w295) -> ()
        n181 = local write "Run Time"(w295) -> ()
        n182 = local write "Downtime"(w295) -> ()
        n183 = local write "Standard DT (Min)"(w295) -> ()
        n184 = local write "Net Avai time (Min)"(w295) -> ()
        n185 = local write "AT time (Min)"(w295) -> ()
        n186 = local write "Rejection Count"(w295) -> ()
      }
    }
    n187 = Unbundle(w125) -> ("mislanius times shift 1"=w121:T13, "mislanius times shift 2"=w122:T13)  [unwired: 6 out]
    n188 = local write "mislanius times shift 2"(w122) -> ()
    n189 = local write "mislanius times shift 1"(w121) -> ()
    n190 = call <vilib>:"Simple Error Handler.vi"("type of dialog (OK msg:1)"=w118, "error in (no error)"=w120) -> ("error out"=w119:errorcluster)  [unwired: 3 in, 4 out]
  }
  n191 = Unbundle By Name(w83) -> ("connection reference"=w82:T8)
  n192 = call <vilib>:"Clear Errors.vi"("error in (no error)"=w2) -> ("error out"=w1:errorcluster)  [unwired: 5 in, 1 out]
  n193 = call <vilib>:"DB Tools Close Connection.vi"("error in (no error)"=w1, "connection reference"=w82) -> ("error out"=w85:errorcluster)  [unwired: 5 in]
  n194 = call <vilib>:"Clear Errors.vi"("error in (no error)"=w85) -> ("error out"=w84:errorcluster)  [unwired: 5 in, 1 out]
  n195 = property class="App"(error in=w84) -> (error out=w87:errorcluster, "App.Kind"=w88:T9)  [unwired: 1 in, 1 out]
  n196 = case shown="\"Run Time System\"" w88 {
    tunnel: w87 -> [w306 w308]
    tunnel: [w306 w307] -> w86
    frame Default {
    }
    frame "Run Time System" {
      n197 = invoke class="VI" method="FP.Close"(error in=w308) -> (error out=w307:errorcluster)  [unwired: 2 in, 2 out]
    }
  }
  "error out 2" <- w86
